vi "LIN EX Ctrl Power Out.vi"(8 "error in (no error)":errorcluster, 10 "State":u8, 11 "DevHandle":i32) -> (0 "error out":errorcluster, 3 "function return":i32)   [LabVIEW 2010, in "usb2lin_ex.lvlib"]
doc: "int WINAPI LIN_EX_CtrlPowerOut(int DevHandle,unsigned char State);"
uses:
  usb2lin_ex.lvlib
  USB2XXX.dll
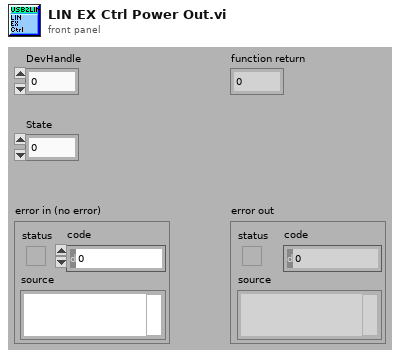
[diagram p1: front panel]
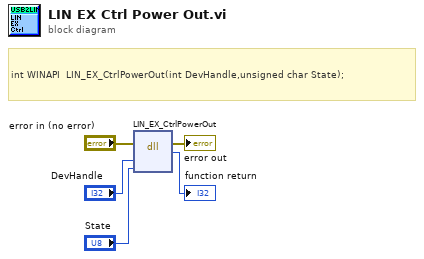
[diagram p0: block diagram]
diagram:
  # "int WINAPI  LIN_EX_CtrlPowerOut(int DevHandle,unsigned char State);"
  n1 = dll-call lib="E:/OtherWork/STM32/USB2XXX_Example/sdk/api/Labview/USB2XXX.*" fn="LIN_EX_CtrlPowerOut"(error in="error in (no error)", "DevHandle"="DevHandle", "State"="State") -> (error out=→"error out":errorcluster, →"function return":i32)  [unwired: 4 in, 1 out]
